vi "PMT_plus_Kinesis_plus_Keithley.vi"() -> ()   [LabVIEW 2022 SP3]
uses:
  <vilib>/Utility/file.llb/Write Delimited Spreadsheet (string).vi
  <vilib>/Analysis/1siggen.llb/Ramp Pattern by Delta.vi
  <vilib>/Utility/file.llb/Write Delimited Spreadsheet (DBL).vi
  C:/Users/Public/OneDrive/Desktop/PMT program/SampleCodeLabView/Kinesis_with_LabVIEW_Examples_LV12 - v3/ThorLabs.MotionControl.KCube.DCServoCLI.dll
  Kinesis_with_LabVIEW_Examples_LV12 - v3/ThorLabs.MotionControl.KCube.DCServoCLI.dll
  <vilib>/Analysis/NI_AALBase.lvlib
  C:/Users/Public/OneDrive/Desktop/PMT program/SampleCodeLabView/Kinesis_with_LabVIEW_Examples_LV12 - v3/Thorlabs.MotionControl.Controls.dll
  Kinesis_with_LabVIEW_Examples_LV12 - v3/Thorlabs.MotionControl.Controls.dll
  test_save_lv22/Close.vi/Close Folder/Users/Public/OneDrive/Desktop/Keithley_2450_2470_1_4_0_LV2015_NewReadme2_2450-LV2015-1.4.0/Keithley 2450/Keithley 2450.lvlib
panel:
  out "XY Graph":cluster{dbl[], dbl[]}(graph)
  out "mean":dbl=49.0
  out "standard deviation":dbl
  out "OLD":bool
  out "data":u32[](array[numeric])=[49, 49]
  out "Actual Voltage 2450":dbl
  out "current 2450":dbl=2.5622937e-12 format="%e"
  out "error out":errorcluster
  out "Set Voltage 2450":dbl
  in  "VISA resource name":refnum<visa-resource-name>="GPIB0::1::INSTR"
  in  "error in (no error)":errorcluster
  out "Serial Configuration":T1={"Baud Rate"=9600, "Parity"=0, "Data Bits"=8, "Stop Bits"=10, "Flow Control"=0} {"Flow Control" items=["None", "XON/XOFF", "RTS/CTS", "XON/XOFF & RTS/CTS", "DTR/DSR", "XON/XOFF & DTR/DSR"]; "Stop Bits" items=["1.0"=10, "1.5"=15, "2.0"=20]; "Data Bits" items=["7"=7, "8"=8]; "Parity" items=["None", "Odd", "Even", "Mark", "Space"]; "Baud Rate" items=["300"=300, "600"=600, "1200"=1200, "2400"=2400, "4800"=4800, "9600"=9600, "19200"=19200]}
  in  "Num Current Meas":i32=20
  in  "Source Limit Level (0.1)":dbl=1e-08
  in  "wait for move (ms)":u32=2000
  out "Handle Number":i32=173123648
  in  "Start V":dbl format="%#_13g"
  in  "End V":dbl=1.0 format="%#_13g"
  in  "Step Size (V)":dbl=0.5 format="%#_13g"
  in  "Path":path=path "C:/Users/Public/OneDrive/Desktop/test.txt"
  in  "Use PMT?":bool=TRUE
  in  "Loop?":bool
  in  "KCubeDCServoControl":refnum<k24>(container)
  in  "Motor Controller\nSerialNumber":string="27268499"
  in  "quarter waveplate p1":dbl=131.0 format="%#_13g"
  in  "quarter waveplate p2":dbl=221.0 format="%#_13g"
  out "PC":dbl caption="Current Rotation Position"
  out "DB":u32[](array[numeric])=[49, 0, 0, 0, 0, 0, 0, 0, 0, 0, 0, 0, 0, 0, 0, 0]
  out "Overload":i32
  out "Gate Number":i32=1
  out "Num Gates Read":i32=2
  out "Gate Time Read":i32=100 caption="Gate time Read"
  out "Num Gates Set":i32=2
  out "Gate Time Set":i32=100
  out "PowerD":i32 caption="Power\nRead Data"
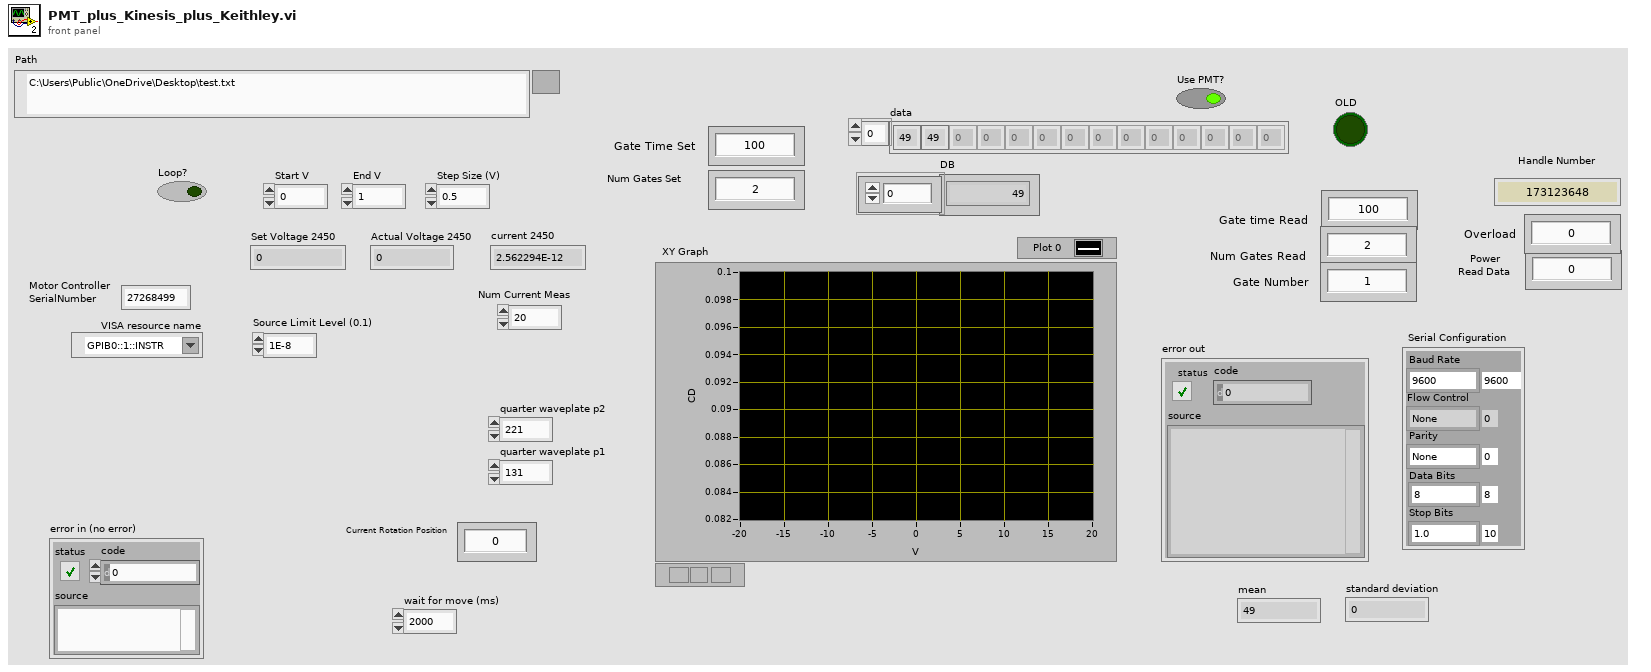
[diagram p1: front panel]
types:
  T1 = cluster{"Baud Rate":u32, "Parity":u16, "Data Bits":u16, "Stop Bits":u16, "Flow Control":u16}
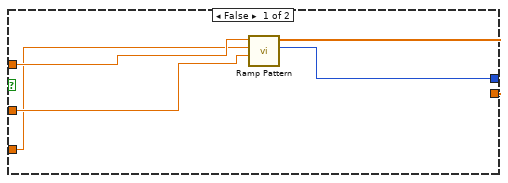
[diagram p2: hidden frame]
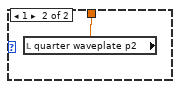
[diagram p3: hidden frame]
diagram:
  n1 = flat-sequence {
    tunnel: [w46] -> w21
    tunnel: [w37] -> w20
    tunnel: ["Path"] -> w19
    tunnel: [w36] -> w18
    tunnel: [w25] -> w17
    tunnel: [w22] -> w16
    tunnel: w21 -> [w82]
    tunnel: [w82] -> w15
    tunnel: w20 -> [w81]
    tunnel: [w81] -> w14
    tunnel: w19 -> [w80]
    tunnel: [w80] -> w13
    tunnel: w18 -> [w79]
    tunnel: [w79] -> w12
    tunnel: [w78] -> w11
    tunnel: w17 -> [w78]
    tunnel: ["wait for move (ms)"] -> w10
    tunnel: [w76] -> w9
    tunnel: w16 -> [w76]
    tunnel: w15 -> [w93]
    tunnel: [w93] -> w8
    tunnel: w14 -> [w92]
    tunnel: [w92] -> w7
    tunnel: w13 -> [w91]
    tunnel: [w91] -> w6
    tunnel: w12 -> [w90]
    tunnel: [w90] -> w5
    tunnel: w11 -> [w89]
    tunnel: [w88] -> w4
    tunnel: [w84] -> w3
    tunnel: w10 -> [w84]
    tunnel: [w83] -> w2
    tunnel: w9 -> [w83]
    tunnel: w8 -> [w105]
    tunnel: w7 -> [w104]
    tunnel: [w103] -> w1
    tunnel: w6 -> [w102]
    tunnel: w5 -> [w97]
    tunnel: w4 -> [w96]
    tunnel: w3 -> [w95]
    tunnel: w2 -> [w94]
    tunnel: w1 -> [w583]
    frame #0 {
      # "open PMT and turn on power"
      n2 = local write "quarter waveplate p2"("quarter waveplate p2") -> ()
      n3 = local write "quarter waveplate p1"("quarter waveplate p1") -> ()
      n4 = call "Open.vi"("Serial Number"="30430219") -> ("Handle Number"=w50:i32)  [unwired: 9 in, 1 out]
      "Handle Number" <- w50
      n5 = case shown="True" "Loop?" {
        tunnel: "Start V" -> [w57 w68]
        tunnel: "End V" -> [w56 w66]
        tunnel: [w59 w65] -> w36
        tunnel: [w60 w64] -> w37
        tunnel: "Step Size (V)" -> [w58 w62]
        frame False {
          n6 = call-poly <vilib>:"Ramp Pattern.vi"("start"=w57, "end"=w56, "delta"=w58) -> ("samples"=w60:i32, "Ramp Pattern"=w59:dbl[])  [unwired: 6 in, 1 out]
        }
        frame True {
          w63 = -1.0
          n7 = Multiply(x=w62, y=w63) -> (x*y=w61:dbl)
          n8 = Multiply(x=w66, y=w63) -> (x*y=w67:dbl)
          n9 = call-poly <vilib>:"Ramp Pattern.vi"("start"=w68, "end"=w66, "delta"=w62) -> ("samples"=w72:i32, "Ramp Pattern"=w69:dbl[])  [unwired: 6 in, 1 out]
          n10 = call-poly <vilib>:"Ramp Pattern.vi"("start"=w67, "end"=w68, "delta"=w62) -> ("samples"=w75:i32, "Ramp Pattern"=w71:dbl[])  [unwired: 6 in, 1 out]
          n11 = call-poly <vilib>:"Ramp Pattern.vi"("start"=w66, "end"=w67, "delta"=w61) -> ("samples"=w73:i32, "Ramp Pattern"=w70:dbl[])  [unwired: 6 in, 1 out]
          n12 = Add(x=w72, y=w73) -> (x+y=w74:i32)
          n13 = Build Array (concatenate)(w69, w70, w71) -> (w65:dbl[])
          n14 = Add(x=w74, y=w75) -> (x+y=w64:i32)
        }
      }
      n15 = call "Read HV.vi"("handle"=w50) -> ("HV out"=w49:i32, "handle out"=w53:i32)  [unwired: 8 in, 1 out]
      n16 = Boolean To (0,1)(Boolean="Use PMT?") -> (0, 1=w51:i16)
      n17 = local write "PowerD"(w49) -> ()
      n18 = To Long Integer(number=w51) -> (32bit integer=w52:i32)
      n19 = call "Set HV.vi"("HV"=w52, "handle"=w53) -> ("handle out"=w55:i32)  [unwired: 8 in, 1 out]
      n20 = property class="KCubeDCServoControl"(reference="KCubeDCServoControl", "SerialNumber"="Motor Controller\nSerialNumber") -> (reference out=w35:refnum<k24>)  [unwired: 1 in, 1 out]
      n21 = invoke class="KCubeDCServoControl" method="CreateDevice"(reference=w35) -> (reference out=w32:refnum<k24>)  [unwired: 2 in, 2 out]
      n22 = property class="KCubeDCServoControl"(reference=w32) -> ("Device"=w22:refnum<k24>)  [unwired: 1 in, 2 out]
      n23 = call "Read HV.vi"("handle"=w55) -> ("HV out"=w54:i32, "handle out"=w46:i32)  [unwired: 8 in, 1 out]
      n24 = local write "PowerD"(w54) -> ()
      n25 = invoke class="KCubeDCServo" method="GetPositionCounter"(reference=w22) -> (reference out=w28:refnum<k24>, "GetPositionCounter"=w31:i32)  [unwired: 2 in, 1 out]
      n26 = Divide(x=w31, y=1919.6418578623338) -> (x/y=w29:dbl)
      n27 = local write "PC"(w29) -> ()
      n28 = invoke class="KCubeDCServo" method="SetMoveAbsolutePosition"(reference=w28, "position"="quarter waveplate p1") -> (reference out=w27:refnum<k24>)  [unwired: 2 in, 3 out]
      n29 = invoke class="KCubeDCServo" method="MoveAbsolute"(reference=w27, "waitTimeout"=0) -> (reference out=w25:refnum<k24>)  [unwired: 2 in, 3 out]
      n30 = Build Array("# SetVoltage2450(V) ActualVoltage2450(V) CountsMeancirc1 Countsmeancirc2 CountsStdcirc1 CountsStdcirc2 Current2450(uA) Current2450Std(uA) CircularDichroism") -> (w41:string[])
      n31 = call-poly <vilib>:"Write Delimited Spreadsheet.vi"("file path (dialog if empty)"="Path", "1D data"=w41, "append to file? (new file:F)"=TRUE) -> ()  [unwired: 11 in, 2 out]
    }
    frame #1 {
      n32 = Wait (ms)(milliseconds to wait="wait for move (ms)") -> ()  [unwired: 1 out]
    }
    frame #2 {
      n33 = invoke class="KCubeDCServo" method="GetPositionCounter"(reference=w89) -> (reference out=w88:refnum<k24>, "GetPositionCounter"=w86:i32)  [unwired: 2 in, 1 out]
      n34 = Divide(x=w86, y=1919.6418578623338) -> (x/y=w85:dbl)
      n35 = local write "PC"(w85) -> ()
    }
    frame #3 {
      w100 = 0
      w101 = 0
      n36 = Initialize Array(w101, w101) -> (w98:i32[])
      n37 = Initialize Array(w100, w100) -> (w99:i32[])
      n38 = for {
        N: w104 -> [_]
        tunnel: w97 -> [w159] mode=indexing
        tunnel: w105 -> [w135]
        tunnel: [w158] -> w103
        tunnel: w102 -> [w131]
        shift-right: [w149] -> _
        shift-left: w98 -> [w154]
        shift-right: [w150] -> _
        shift-left: w99 -> [w153]
        tunnel: w96 -> [w127]
        tunnel: w95 -> [w123]
        tunnel: w94 -> [w109]
        n39 = flat-sequence {
          tunnel: w153 -> [w193]
          tunnel: w154 -> [w194]
          tunnel: w159 -> [w189]
          tunnel: [w189] -> w148
          tunnel: [w194] -> w146
          tunnel: [w193] -> w144
          tunnel: [w192] -> w142
          tunnel: [w191] -> w140
          tunnel: ["Num Current Meas"] -> w136
          tunnel: w135 -> [w169]
          tunnel: [w169] -> w132
          tunnel: w131 -> [w168]
          tunnel: [w168] -> w128
          tunnel: w127 -> [w167]
          tunnel: [w167] -> w124
          tunnel: w109 -> [w166]
          tunnel: [w166] -> w107
          tunnel: w148 -> [w205]
          tunnel: [w205] -> w147
          tunnel: w146 -> [w204]
          tunnel: [w204] -> w145
          tunnel: w144 -> [w203]
          tunnel: [w203] -> w143
          tunnel: w142 -> [w202]
          tunnel: [w202] -> w141
          tunnel: w140 -> [w201]
          tunnel: [w201] -> w139
          tunnel: [w200] -> w137
          tunnel: w136 -> [w200]
          tunnel: [w198] -> w133
          tunnel: w132 -> [w198]
          tunnel: [w197] -> w129
          tunnel: w128 -> [w197]
          tunnel: [w196] -> w125
          tunnel: w124 -> [w196]
          tunnel: [w195] -> w108
          tunnel: w107 -> [w195]
          tunnel: [w236] -> w157
          tunnel: [w237] -> w156
          tunnel: [w229] -> w155
          tunnel: [w235] -> w152
          tunnel: [w234] -> w151
          tunnel: w147 -> [w236]
          tunnel: w145 -> [w235]
          tunnel: w143 -> [w234]
          tunnel: w141 -> [w232]
          tunnel: w139 -> [w233]
          tunnel: [w230] -> w138
          tunnel: w137 -> [w231]
          tunnel: [w209] -> w134
          tunnel: w133 -> [w209]
          tunnel: [w208] -> w130
          tunnel: w129 -> [w208]
          tunnel: [w207] -> w126
          tunnel: w125 -> [w207]
          tunnel: w108 -> [w206]
          tunnel: [w206] -> w106
          tunnel: w157 -> [w261]
          tunnel: w156 -> [w260]
          tunnel: w155 -> [w259]
          tunnel: w152 -> [w258]
          tunnel: w151 -> [w257]
          tunnel: [w262] -> w122
          tunnel: [w256] -> w119
          tunnel: w138 -> [w255]
          tunnel: w134 -> [w254]
          tunnel: w130 -> [w250]
          tunnel: w126 -> [w252]
          tunnel: w123 -> [w251]
          tunnel: [w250] -> w117
          tunnel: [w249] -> w116
          tunnel: [w244] -> w115
          tunnel: [w243] -> w114
          tunnel: [w242] -> w113
          tunnel: [w241] -> w112
          tunnel: [w240] -> w111
          tunnel: [w239] -> w110
          tunnel: w106 -> [w238]
          tunnel: w122 -> [w578]
          tunnel: [w578] -> w121
          tunnel: [w569] -> w120
          tunnel: w119 -> [w560]
          tunnel: [w559] -> w118
          tunnel: w117 -> [w576]
          tunnel: w116 -> [w574]
          tunnel: w115 -> [w557]
          tunnel: w114 -> [w567]
          tunnel: w113 -> [w573]
          tunnel: w112 -> [w572]
          tunnel: w111 -> [w570]
          tunnel: w110 -> [w568]
          tunnel: [w580] -> w149
          tunnel: [w581] -> w150
          tunnel: [w582] -> w158
          tunnel: w121 -> [w582]
          tunnel: w120 -> [w581]
          tunnel: w118 -> [w580]
          frame #0 {
            w176 = 1
            w178 = 0
            w187 = TRUE
            n40 = call "Initialize.vi"("error in (no error)"="error in (no error)", "Reset (True)"=FALSE, "ID Query (True)"=TRUE, "VISA resource name"="VISA resource name") -> ("error out"=w160:errorcluster, "VISA resource name out"=w165:refnum<visa-resource-name>)  [unwired: 6 in]
            n41 = call "Clear Buffer.vi"("VISA resource name"=w165, "error in (no error)"=w160) -> ("VISA resource name out"=w174:refnum<visa-resource-name>, "error out"=w175:errorcluster)  [unwired: 12 in]
            n42 = call "Configure Measurement Range.vi"("error in (no error)"=w175, "Enable Auto Range (T:Enable)"=w187, "Function (0: Volts)"=w178, "VISA resource name"=w174) -> ("error out"=w186:errorcluster, "VISA resource name out"=w185:refnum<visa-resource-name>)  [unwired: 6 in]
            n43 = call "Configure Measurement Range.vi"("error in (no error)"=w186, "Enable Auto Range (T:Enable)"=w187, "Function (0: Volts)"=w176, "VISA resource name"=w185) -> ("error out"=w182:errorcluster, "VISA resource name out"=w179:refnum<visa-resource-name>)  [unwired: 6 in]
            n44 = call "Configure Output.vi"("VISA resource name"=w179, "Source Level (0)"=w189, "Source Limit Level (0.1)"="Source Limit Level (0.1)", "error in (no error)"=w182) -> ("VISA resource name out"=w180:refnum<visa-resource-name>, "error out"=w183:errorcluster)  [unwired: 10 in]
            n45 = call "Configure Source Function.vi"("error in (no error)"=w183, "Function (0: Volts)"=w178, "VISA resource name"=w180) -> ("error out"=w184:errorcluster, "VISA resource name out"=w181:refnum<visa-resource-name>)  [unwired: 7 in]
            n46 = call "Configure Measurement Function.vi"("error in (no error)"=w184, "Function (0: Volts)"=w176, "VISA resource name"=w181) -> ("error out"=w170:errorcluster, "VISA resource name out"=w173:refnum<visa-resource-name>)  [unwired: 7 in]
            n47 = call "Set Measurement Count.vi"("error in (no error)"=w170, "Measurement Count (1)"="Num Current Meas", "VISA resource name"=w173) -> ("error out"=w171:errorcluster, "VISA resource name out"=w172:refnum<visa-resource-name>)  [unwired: 7 in]
            n48 = call "Enable Output.vi"("error in (no error)"=w171, "Enable Output (T: Enable)"=TRUE, "VISA resource name"=w172) -> ("error out"=w192:errorcluster, "VISA resource name out"=w191:refnum<visa-resource-name>)  [unwired: 7 in]
            "Set Voltage 2450" <- w189
          }
          frame #1 {
            n49 = Wait (ms)(milliseconds to wait=u32 100) -> ()  [unwired: 1 out]
          }
          frame #2 {
            w213 = 1000000
            n50 = call "Make Reading and Store in Buffer.vi"("VISA resource name"=w233, "error in (no error)"=w232) -> ("VISA resource name out"=w225:refnum<visa-resource-name>, "error out"=w224:errorcluster)  [unwired: 12 in]
            n51 = call "Read (Multiple Points).vi"("VISA resource name"=w225, "Start Index (1)"=u32 1, "End Index (1)"=w231, "error in (no error)"=w224) -> ("VISA resource name out"=w217:refnum<visa-resource-name>, "Data out"=w222:string, "error out"=w216:errorcluster)  [unwired: 9 in]
            n52 = call "Get Source Level.vi"("error in (no error)"=w216, "VISA resource name"=w217) -> ("error out"=w227:errorcluster, "Voltage Level Out"=w237:dbl, "VISA resource name out"=w228:refnum<visa-resource-name>)  [unwired: 6 in, 1 out]
            "Actual Voltage 2450" <- w237
            n53 = Spreadsheet String To Array(delimiter (Tab)=",", format string="%s", spreadsheet string=w222, array type (2D Dbl)=dbl[] []) -> (array=w218:dbl[])
            n54 = call "Enable Output.vi"("error in (no error)"=w227, "Enable Output (T: Enable)"=TRUE, "VISA resource name"=w228) -> ("error out"=w210:errorcluster, "VISA resource name out"=w211:refnum<visa-resource-name>)  [unwired: 7 in]
            n55 = call "Close.vi"("error in (no error)"=w210, "VISA resource name"=w211) -> ("error out"=→"error out":errorcluster)  [unwired: 9 in]
            n56 = call <vilib>:"Std Deviation and Variance.vi"("X"=w218) -> ("mean"=w214:dbl, "standard deviation"=w215:dbl)  [unwired: 1 in, 1 out]
            "current 2450" <- w214
            n57 = Multiply(x=w215, y=w213) -> (x*y=w230:dbl)
            n58 = Multiply(x=w214, y=w213) -> (x*y=w229:dbl)
          }
          frame #3 {
            w246 = 0
            w248 = 0
            n59 = Initialize Array(w248, w248) -> (w247:i32[])
            n60 = Initialize Array(w246, w246) -> (w245:i32[])
            n61 = for {
              N: 2 -> [_]
              tunnel: w261 -> [w372]
              tunnel: w260 -> [w371]
              tunnel: w259 -> [w370]
              tunnel: w258 -> [w292]
              tunnel: w257 -> [w369]
              tunnel: [w368] -> w256
              tunnel: w255 -> [w367]
              shift-right: [w373] -> w262
              shift-left: w254 -> [w366]
              tunnel: w252 -> [w304]
              tunnel: w251 -> [w303]
              tunnel: [w293] -> w249
              shift-right: [w271] -> w244
              shift-left: w247 -> [w291]
              shift-right: [w270] -> w243
              shift-left: w245 -> [w281]
              tunnel: [w269] -> w242
              tunnel: [w268] -> w241
              tunnel: [w267] -> w240
              tunnel: [w266] -> w239
              tunnel: w238 -> [w265]
              i -> [w302]
              (unwired) "# SetVoltage2450(V) ActualVoltage2450(V) CountsMean CountsStd Current2450(uA) Current2450Std(uA)"
              # "- actual voltage array\n- actual voltage current\n- set voltage current\n-  current current\n- current std current"
              n62 = flat-sequence {
                tunnel: [w385] -> w318
                tunnel: [w383] -> w316
                tunnel: [w384] -> w314
                tunnel: w372 -> [w385]
                tunnel: w371 -> [w384]
                tunnel: w370 -> [w383]
                tunnel: w292 -> [w382]
                tunnel: [w382] -> w312
                tunnel: w369 -> [w381]
                tunnel: [w381] -> w310
                tunnel: w367 -> [w380]
                tunnel: [w380] -> w308
                tunnel: w366 -> [w379]
                tunnel: [w379] -> w306
                tunnel: w304 -> [_]
                tunnel: w302 -> [w377]
                tunnel: w291 -> [w376]
                tunnel: [w376] -> w287
                tunnel: w281 -> [w375]
                tunnel: [w375] -> w274
                tunnel: w265 -> [w374]
                tunnel: [w374] -> w264
                tunnel: w318 -> [w399]
                tunnel: [w399] -> w317
                tunnel: w316 -> [w398]
                tunnel: [w398] -> w315
                tunnel: w314 -> [w397]
                tunnel: [w397] -> w313
                tunnel: w312 -> [w396]
                tunnel: [w396] -> w311
                tunnel: w310 -> [w395]
                tunnel: [w395] -> w309
                tunnel: w308 -> [w394]
                tunnel: [w394] -> w307
                tunnel: w306 -> [w393]
                tunnel: [w393] -> w305
                tunnel: [w391] -> w288
                tunnel: w287 -> [w391]
                tunnel: [w390] -> w275
                tunnel: w274 -> [w390]
                tunnel: w264 -> [w389]
                tunnel: [w388] -> w263
                tunnel: [w407] -> w365
                tunnel: [w413] -> w364
                tunnel: w317 -> [w413]
                tunnel: [w412] -> w363
                tunnel: w315 -> [w412]
                tunnel: [w411] -> w362
                tunnel: w313 -> [w411]
                tunnel: [w410] -> w361
                tunnel: w311 -> [w410]
                tunnel: [w409] -> w360
                tunnel: w309 -> [w409]
                tunnel: [w408] -> w359
                tunnel: w307 -> [w408]
                tunnel: w305 -> [w407]
                tunnel: w303 -> [w406]
                tunnel: [w405] -> w289
                tunnel: w288 -> [w405]
                tunnel: [w404] -> w276
                tunnel: w275 -> [w404]
                tunnel: w263 -> [w400]
                tunnel: w365 -> [w428]
                tunnel: [w423] -> w358
                tunnel: [w421] -> w357
                tunnel: w364 -> [w421]
                tunnel: [w420] -> w356
                tunnel: w363 -> [w420]
                tunnel: [w419] -> w355
                tunnel: w362 -> [w419]
                tunnel: [w418] -> w354
                tunnel: w361 -> [w418]
                tunnel: [w417] -> w353
                tunnel: w360 -> [w417]
                tunnel: [w416] -> w352
                tunnel: w359 -> [w416]
                tunnel: [w415] -> w290
                tunnel: w289 -> [w415]
                tunnel: [w414] -> w277
                tunnel: w276 -> [w414]
                tunnel: [w439] -> w351
                tunnel: w358 -> [w441]
                tunnel: [w436] -> w350
                tunnel: w357 -> [w436]
                tunnel: w356 -> [w435]
                tunnel: [w435] -> w349
                tunnel: [w434] -> w348
                tunnel: w355 -> [w434]
                tunnel: [w433] -> w347
                tunnel: w354 -> [w433]
                tunnel: [w432] -> w346
                tunnel: w353 -> [w432]
                tunnel: [w431] -> w345
                tunnel: w352 -> [w431]
                tunnel: w290 -> [w430]
                tunnel: [w430] -> w284
                tunnel: [w429] -> w278
                tunnel: w277 -> [w429]
                tunnel: w351 -> [w456]
                tunnel: [w456] -> w344
                tunnel: [w452] -> w343
                tunnel: [w452] -> w342
                tunnel: [w451] -> w341
                tunnel: w350 -> [w451]
                tunnel: [w450] -> w340
                tunnel: w349 -> [w450]
                tunnel: w348 -> [w449]
                tunnel: [w449] -> w339
                tunnel: [w448] -> w338
                tunnel: w347 -> [w448]
                tunnel: [w447] -> w337
                tunnel: w346 -> [w447]
                tunnel: w345 -> [w446]
                tunnel: [w446] -> w336
                tunnel: [w445] -> w285
                tunnel: w284 -> [w445]
                tunnel: [w444] -> w279
                tunnel: w278 -> [w444]
                tunnel: w344 -> [w471]
                tunnel: [w467] -> w335
                tunnel: w343 -> [w466]
                tunnel: w342 -> [w465]
                tunnel: [w466] -> w334
                tunnel: [w465] -> w333
                tunnel: w341 -> [w464]
                tunnel: [w464] -> w332
                tunnel: [w463] -> w331
                tunnel: w340 -> [w463]
                tunnel: [w462] -> w330
                tunnel: w339 -> [w462]
                tunnel: [w461] -> w329
                tunnel: w338 -> [w461]
                tunnel: [w460] -> w328
                tunnel: w337 -> [w460]
                tunnel: [w459] -> w327
                tunnel: w336 -> [w459]
                tunnel: [w458] -> w286
                tunnel: w285 -> [w458]
                tunnel: [w457] -> w280
                tunnel: w279 -> [w457]
                tunnel: [w486] -> w326
                tunnel: w335 -> [w485]
                tunnel: w334 -> [w484]
                tunnel: w333 -> [w483]
                tunnel: [w482] -> w325
                tunnel: [w479] -> w324
                tunnel: w332 -> [w479]
                tunnel: [w478] -> w323
                tunnel: w331 -> [w478]
                tunnel: w330 -> [w477]
                tunnel: [w477] -> w322
                tunnel: [w476] -> w321
                tunnel: w329 -> [w476]
                tunnel: [w475] -> w320
                tunnel: w328 -> [w475]
                tunnel: [w474] -> w319
                tunnel: w327 -> [w474]
                tunnel: w286 -> [w473]
                tunnel: [w473] -> w283
                tunnel: w280 -> [w472]
                tunnel: [w472] -> w273
                tunnel: w326 -> [w542]
                tunnel: [w541] -> w300
                tunnel: [w540] -> w301
                tunnel: w325 -> [w540]
                tunnel: w324 -> [w539]
                tunnel: [w539] -> w299
                tunnel: [w538] -> w298
                tunnel: w323 -> [w538]
                tunnel: [w537] -> w297
                tunnel: w322 -> [w537]
                tunnel: [w536] -> w296
                tunnel: w321 -> [w536]
                tunnel: w320 -> [w535]
                tunnel: [w535] -> w295
                tunnel: [w534] -> w294
                tunnel: w319 -> [w534]
                tunnel: w283 -> [w533]
                tunnel: [w533] -> w282
                tunnel: w273 -> [w532]
                tunnel: [w532] -> w272
                tunnel: [w556] -> w373
                tunnel: w300 -> [w556]
                tunnel: w299 -> [w554]
                tunnel: w298 -> [w548]
                tunnel: w297 -> [w546]
                tunnel: w296 -> [w543]
                tunnel: w295 -> [w547]
                tunnel: [w543] -> w368
                tunnel: w294 -> [w545]
                tunnel: w301 -> [w555]
                tunnel: [w554] -> w293
                tunnel: w282 -> [w553]
                tunnel: w272 -> [w552]
                tunnel: [w550] -> w271
                tunnel: [w549] -> w270
                tunnel: [w548] -> w269
                tunnel: [w545] -> w268
                tunnel: [w547] -> w267
                tunnel: [w546] -> w266
                frame #0 {
                  n63 = case shown="0, Default" w377 {
                    tunnel: [w386 w387] -> w378
                    frame 0, Default {
                      n64 = local read "quarter waveplate p1"() -> (w386:dbl)
                    }
                    frame 1 {
                      n65 = local read "quarter waveplate p2"() -> (w387:dbl)
                    }
                  }
                  n66 = invoke class="KCubeDCServo" method="SetMoveAbsolutePosition"(reference=w374, "position"=w378) -> ()  [unwired: 2 in, 4 out]
                }
                frame #1 {
                  n67 = invoke class="KCubeDCServo" method="MoveAbsolute"(reference=w389, "waitTimeout"=0) -> (reference out=w388:refnum<k24>)  [unwired: 2 in, 3 out]
                }
                frame #2 {
                  n68 = Wait (ms)(milliseconds to wait=w406) -> ()  [unwired: 1 out]
                  n69 = invoke class="KCubeDCServo" method="GetPositionCounter"(reference=w400) -> ("GetPositionCounter"=w402:i32)  [unwired: 2 in, 2 out]
                  n70 = Divide(x=w402, y=1919.6418578623338) -> (x/y=w401:dbl)
                  n71 = local write "PC"(w401) -> ()
                }
                frame #3 {
                  # "set gate time"
                  n72 = local read "Gate Time Set"() -> (w425:i32)
                  n73 = Wait (ms)(milliseconds to wait=u32 200) -> ()  [unwired: 1 out]
                  n74 = To Long Integer(number=w425) -> (32bit integer=w426:i32)
                  n75 = call "Set IT.vi"("IT"=w426, "handle"=w428) -> ("handle out"=w427:i32)  [unwired: 8 in, 1 out]
                  n76 = call "Read IT.vi"("handle"=w427) -> ("IT out"=w424:i32, "handle out"=w423:i32)  [unwired: 8 in, 1 out]
                  n77 = local write "Gate Time Read"(w424) -> ()
                }
                frame #4 {
                  # "set number of gates"
                  n78 = local read "Num Gates Set"() -> (w443:i32)
                  n79 = Wait (ms)(milliseconds to wait=u32 200) -> ()  [unwired: 1 out]
                  n80 = To Long Integer(number=w443) -> (32bit integer=w442:i32)
                  n81 = call "Set RN.vi"("RN"=w442, "handle"=w441) -> ("handle out"=w440:i32)  [unwired: 8 in, 1 out]
                  n82 = call "Read RN.vi"("handle"=w440) -> ("RN out"=w438:i32, "handle out"=w439:i32)  [unwired: 8 in, 1 out]
                  n83 = local write "Num Gates Read"(w438) -> ()
                }
                frame #5 {
                  # "gate number data"
                  # "count data"
                  n84 = local write "Gate Number"(0) -> ()
                  n85 = Initialize Array(u32 0, 0 ("次元サイズ")) -> (w452:u32[])
                }
                frame #6 {
                  n86 = Boolean To (0,1)(Boolean=TRUE ("Correction")) -> (0, 1=w470:i16)
                  n87 = To Long Integer(number=w470) -> (32bit integer=w469:i32)
                  n88 = call "Count Start.vi"("Correction"=w469, "handle"=w471) -> ("handle out"=w467:i32)  [unwired: 8 in, 1 out]
                }
                frame #7 {
                  n89 = local read "Num Gates Read"() -> (w481:i32)
                  n90 = for {
                    N: w481 -> [_]
                    shift-right: [w487] -> w482
                    shift-left: w484 -> [w495]
                    shift-right: [w491] -> _
                    shift-left: w483 -> [w494]
                    tunnel: w485 -> [w496]
                    tunnel: [w497] -> w486
                    tunnel: [w487] -> w480
                    n91 = flat-sequence {
                      tunnel: [w507] -> w501
                      tunnel: [w506] -> w492
                      tunnel: [w505] -> w489
                      tunnel: w496 -> [w507]
                      tunnel: w495 -> [w506]
                      tunnel: w494 -> [w505]
                      tunnel: [w518] -> w500
                      tunnel: w501 -> [w517]
                      tunnel: [w512] -> w499
                      tunnel: [w511] -> w498
                      tunnel: [w510] -> w493
                      tunnel: w492 -> [w510]
                      tunnel: [w509] -> w490
                      tunnel: w489 -> [w509]
                      tunnel: [w508] -> w488
                      tunnel: w500 -> [w531]
                      tunnel: w499 -> [w526]
                      tunnel: w498 -> [w525]
                      tunnel: w493 -> [w523]
                      tunnel: w490 -> [w522]
                      tunnel: w488 -> [w521]
                      tunnel: [w531] -> w497
                      tunnel: [w524] -> w487
                      tunnel: [w519] -> w491
                      frame #0 {
                        n92 = Initialize Array(u32 0, 16 ("次元サイズ")) -> (w502:u32[])
                        n93 = local write "DB"(w502) -> ()
                      }
                      frame #1 {
                        # "read data"
                        n94 = local read "Gate Number"() -> (w516:i32)
                        n95 = local read "Overload"() -> (w515:i32)
                        n96 = local read "DB"() -> (w513:u32[])
                        n97 = call "Read Data.vi"("OLD"=w515, "DataBuf"=w513, "GateNum"=w516, "handle"=w517) -> ("OLD out"=w514:i32, "DataBuf out"=w511:u32[], "GateNum out"=w508:i32, "handle out"=w518:i32, "function return"=w512:u32)  [unwired: 3 in]
                        n98 = local write "Gate Number"(w508) -> ()
                        n99 = local write "DB"(w511) -> ()
                        n100 = local write "Overload"(w514) -> ()
                      }
                      frame #2 {
                        # "Pickup Tans Data!"
                        n101 = To Long Integer(number=w526) -> (32bit integer=w527:i32)
                        n102 = Build Array(w521) -> (w520:i32[])
                        n103 = local read "Overload"() -> (w529:i32)
                        n104 = Build Array (concatenate)(w522, w520) -> (w519:u32[])
                        n105 = Array Subset(array=w525, length=w527) -> (w528:u32[])  [unwired: 1 in]
                        n106 = Not Equal To 0?(x=w529) -> (x != 0?=→"OLD":bool)
                        n107 = Build Array (concatenate)(w523, w528) -> (w524:u32[])
                      }
                    }
                  }
                  "data" <- w480
                }
                frame #8 {
                  # "data"
                  n108 = call "Count Stop.vi"("handle"=w542) -> ("handle out"=w541:i32)  [unwired: 9 in, 1 out]
                }
                frame #9 {
                  n109 = call <vilib>:"Std Deviation and Variance.vi"("X"=w555) -> ("mean"=w544:dbl, "standard deviation"=w551:dbl)  [unwired: 1 in, 1 out]
                  "mean" <- w544
                  "standard deviation" <- w551
                  n110 = Build Array (concatenate)(w552, w551) -> (w549:dbl[])
                  n111 = Build Array (concatenate)(w553, w544) -> (w550:dbl[])
                }
              }
            }
          }
          frame #4 {
            (unwired) "# SetVoltage2450(V) ActualVoltage2450(V) CountsMeanCirc1 CountsMeanCirc2 CountsStdCirc1 CountsStdCirc2 Current2450(uA) Current2450Std(uA)\nCirculardichroism"
            n112 = Build Array (concatenate)(w570, w568) -> (w569:dbl[])
            n113 = Index Array(array=w557, index=1) -> (element=w563:dbl)
            n114 = Index Array(array=w557, index=0) -> (element=w564:dbl)
            n115 = Subtract(x=w564, y=w563) -> (x-y=w562:dbl)
            n116 = Add(x=w564, y=w563) -> (x+y=w561:dbl)
            n117 = Divide(x=w562, y=w561) -> (x/y=w558:dbl)
            n118 = Build Array (concatenate)(w574, w568, w557, w567, w573, w572, w558) -> (w571:dbl[])
            n119 = call-poly <vilib>:"Write Delimited Spreadsheet.vi"("file path (dialog if empty)"=w576, "format (%.3f)"="%.10f", "1D data"=w571, "append to file? (new file:F)"=TRUE) -> ()  [unwired: 10 in, 2 out]
            n120 = Build Array (concatenate)(w560, w558) -> (w559:dbl[])
          }
          frame #5 {
            n121 = Bundle(w581, w580) -> (→"XY Graph":cluster{dbl[], dbl[]})  [unwired: 1 in]
          }
        }
      }
    }
    frame #4 {
      # "turn off PMT and close"
      n122 = Boolean To (0,1)(Boolean=FALSE) -> (0, 1=w588:i16)
      n123 = To Long Integer(number=w588) -> (32bit integer=w587:i32)
      n124 = call "Set HV.vi"("HV"=w587, "handle"=w583) -> ("handle out"=w585:i32)  [unwired: 8 in, 1 out]
      n125 = call "Read HV.vi"("handle"=w585) -> ("HV out"=w589:i32, "handle out"=w584:i32)  [unwired: 8 in, 1 out]
      n126 = call "Close.vi"("Handle"=w584) -> ()  [unwired: 9 in, 2 out]
      n127 = local write "PowerD"(w589) -> ()
    }
  }
